vi "Initialization_HGB2.vi"(8 "error in":errorcluster, 11 "Sample Rate":dbl=10.0) -> (0 "error out":errorcluster, 3 "Task Array":refnum<k21>[](array[refnum]), 4 "output cluster":T1={"All Channels"=["cDAQ1Mod1/ai0", "cDAQ1Mod1/ai1", "cDAQ1Mod1/ai2", "cDAQ1Mod1/ai3", "cDAQ1Mod1/ai4", "cDAQ1Mod1/ai5", "cDAQ1Mod1/ai6", "cDAQ1Mod1/ai7", "cDAQ1Mod1/ai8", "cDAQ1Mod1/ai9", "cDAQ1Mod1/ai10", "cDAQ1Mod1/ai11", "cDAQ1Mod1/ai12", "cDAQ1Mod1/ai13", "cDAQ1Mod1/ai14", "cDAQ1Mod1/ai15", "cDAQ1Mod2/ai0", "cDAQ1Mod2/ai1", "cDAQ1Mod2/ai2", "cDAQ1Mod2/ai3", "cDAQ1Mod2/ai4", "cDAQ1Mod2/ai5", "cDAQ1Mod2/ai6", "cDAQ1Mod2/ai7", "cDAQ1Mod4/ai0", "cDAQ1Mod4/ai1", "cDAQ1Mod4/ai2", "Dev1/ai0", "Dev1/ai1", "Dev1/ao0", "Dev1/ao1"], "All Labels"=["T_dis", "T_liq_mix", "T_gas_mix", "T_wf_cond_out", "T_cf_in", "NC1", "NC2", "NC3", "NC4", "NC5", "NC6", "NC7", "NC8", "NC9", "NC10", "NC11", "P_comp_suc", "P_comp_dis", "P_comp_int", "m_dot_wf", "Voltage", "Frequency", "NC12", "NC13", "Accel_X", "Accel_Y", "Accel_Z", "Torque", "Tachometer", "Speed Setpoint", "ON-OFF"], "All Units"=["C", "C", "C", "C", "C", "C", "C", "C", "C", "C", "C", "C", "C", "C", "C", "C", "kPa", "kPa", "kPa", "kg/s", "V", "Hz", "A", "A", "g", "g", "g", "N-m", "RPM", "V", "V"], "Slope"=[1.0, 1.0, 1.0, 1.0, 1.0, 1.0, 1.0, 1.0, 1.0, 1.0, 1.0, 1.0, 1.0, 1.0, 1.0, 1.0, 129276.875, 129276.875, 129276.875, 4.6875, 18750.0, 6250.0, 5.0, 6250.0, 1.0, 1.0, 1.0, 4.0, 1600.0, 1.0, 1.0], "Y-Intercept"=[0.0, 0.0, 0.0, 0.0, 0.0, 0.0, 0.0, 0.0, 0.0, 0.0, 0.0, 0.0, 0.0, 0.0, 0.0, 0.0, -432.107, -435.107, -432.107, -0.01875, -75.0, -25.0, 0.0, 0.0, 0.0, 0.0, 0.0, 0.0, 0.0, 0.0, 0.0]})   [LabVIEW 2016]
uses:
  <vilib>/Utility/error.llb/DialogType.ctl
  <vilib>/DAQmx/create/channels.llb/DAQmx Create Channel (AI-Temperature-Thermocouple).vi
  <vilib>/DAQmx/create/scale.llb/DAQmx Create Scale (Linear).vi
  <vilib>/DAQmx/create/channels.llb/DAQmx Create Channel (AI-Voltage-Basic).vi
  <vilib>/DAQmx/create/channels.llb/DAQmx Create Channel (AO-Voltage-Basic).vi
  <vilib>/DAQmx/create/channels.llb/DAQmx Create Channel (AI-Current-Basic).vi
  <vilib>/DAQmx/create/channels.llb/DAQmx Create Channel (AO-Current-Basic).vi
  <vilib>/DAQmx/create/channels.llb/DAQmx Create Channel (AI-Acceleration-Accelerometer).vi
  <vilib>/DAQmx/configure/timing.llb/DAQmx Timing (Sample Clock).vi
panel:
  in  "Tab Control":enum32{"User Inputs", "Sub VI I/O"}(tab)
  in  "All Units":string[](array[string])=["C", "C", "C", "C", "C", "C", "C", "C", "C", "C", "C", "C", "C", "C", "C", "C", "Hz", "V", "kPa", "kPa", "kPa", "kg/s", "A", "A", "g", "g", "g", "N-m", "RPM", "V", "V"]
  in  "Number/Types of Channels per Task":string[][](table)=[["16", "0", "0", "0"], ["0", "0", "2", "0"], ["0", "0", "0", "2"], ["8", "0", "0", "0"], ["0", "0", "0", ""], ["0", "3", "0", ""], ["0", "0", "0", ""]]
  in  "All Channels":tag[](array[tag])=["cDAQ1Mod1/ai0", "cDAQ1Mod1/ai1", "cDAQ1Mod1/ai2", "cDAQ1Mod1/ai3", "cDAQ1Mod1/ai4", "cDAQ1Mod1/ai5", "cDAQ1Mod1/ai6", "cDAQ1Mod1/ai7", "cDAQ1Mod1/ai8", "cDAQ1Mod1/ai9", "cDAQ1Mod1/ai10", "cDAQ1Mod1/ai11", "cDAQ1Mod1/ai12", "cDAQ1Mod1/ai13", "cDAQ1Mod1/ai14", "cDAQ1Mod1/ai15", "cDAQ1Mod2/ai0", "cDAQ1Mod2/ai1", "cDAQ1Mod2/ai2", "cDAQ1Mod2/ai3", "cDAQ1Mod2/ai4", "cDAQ1Mod2/ai5", "cDAQ1Mod2/ai6", "cDAQ1Mod2/ai7", "cDAQ1Mod4/ai0", "cDAQ1Mod4/ai1", "cDAQ1Mod4/ai2", "Dev1/ai0", "Dev1/ai1", "Dev1/ao0", "Dev1/ao1"]
  in  "Task Count":i32=4
  in  "All Labels":string[](array[string])=["T_comp_suc", "T_comp_out", "NC1", "T_gas_mix", "T_wf_cd_out", "T_liq", "T_cf_in", "T_dis_dwnstrm", "NC2", "NC3", "NC4", "NC5", "NC6", "NC7", "NC8", "NC9", "Frequency", "Voltage", "P_comp_suc", "P_comp_dis", "P_comp_int", "m_dot_wf", "NC12", "NC13", "Accel_X", "Accel_Y", "Accel_Z", "Torque", "Tachometer", "Speed Setpoint", "ON-OFF"]
  in  "Y-Intercept":dbl[](array[numeric])=[0.0, 0.0, 0.0, 0.0, 0.0, 0.0, 0.0, 0.0, 0.0, 0.0, 0.0, 0.0, 0.0, 0.0, 0.0, 0.0, -25.0, -75.0, -432.107, -432.107, -432.107, -0.0225, 0.0, 0.0, 0.0, 0.0, 0.0, 0.0, 0.0, 0.0, 0.0]
  in  "Slope":dbl[](array[numeric])=[1.0, 1.0, 1.0, 1.0, 1.0, 1.0, 1.0, 1.0, 1.0, 1.0, 1.0, 1.0, 1.0, 1.0, 1.0, 1.0, 6250.0, 18750.0, 129276.875, 129277.0, 129277.0, 5.625, 5.0, 6250.0, 1.0, 1.0, 1.0, 4.0, 1600.0, 1.0, 1.0]
  # "*Make Current Values Default and Save Before Closing Sub VI*"
  # "*List the read and write channels of any hardware as separate devices*"
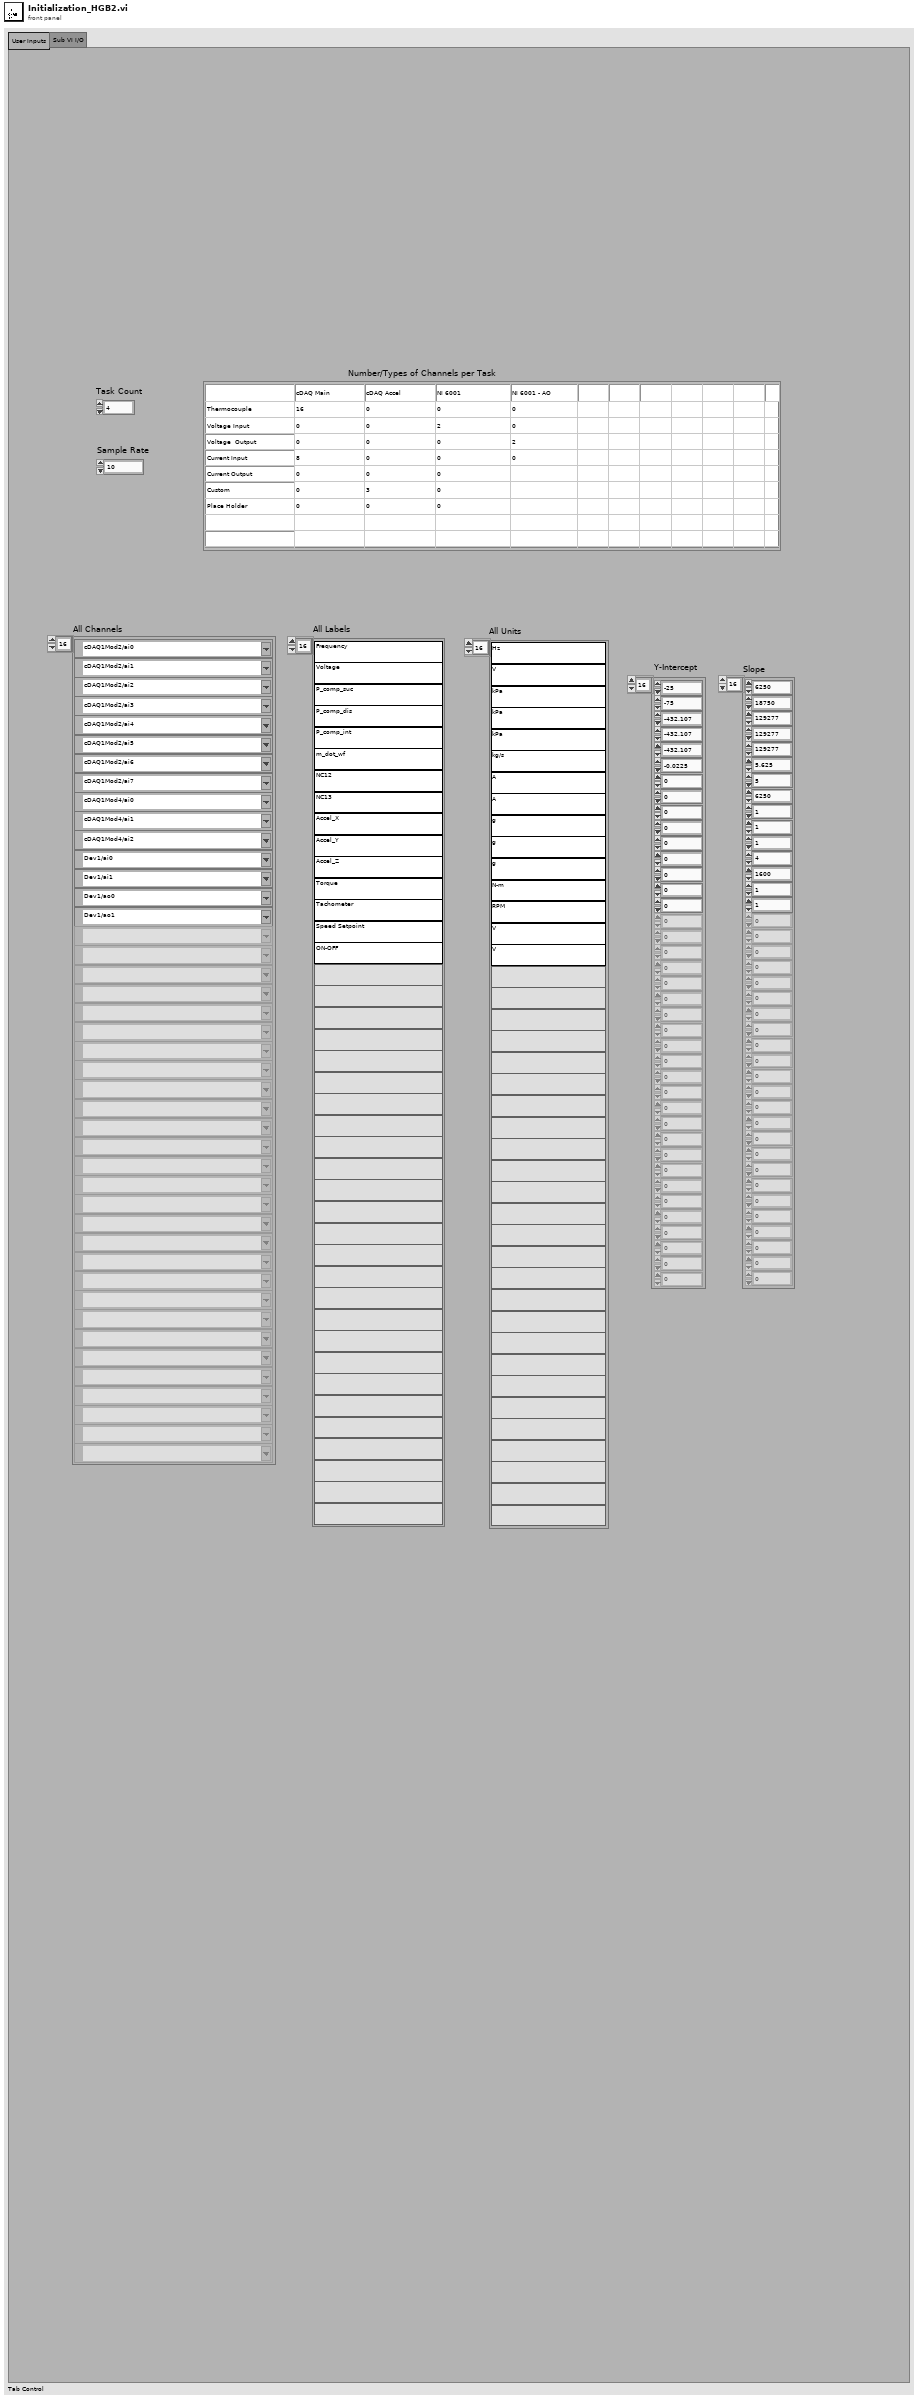
[diagram p1: front panel]
types:
  T1 = cluster{"All Channels":tag[], "All Labels":string[], "All Units":string[], "Slope":dbl[], "Y-Intercept":dbl[]}
  T2 = typedef "DialogType.ctl" = u16
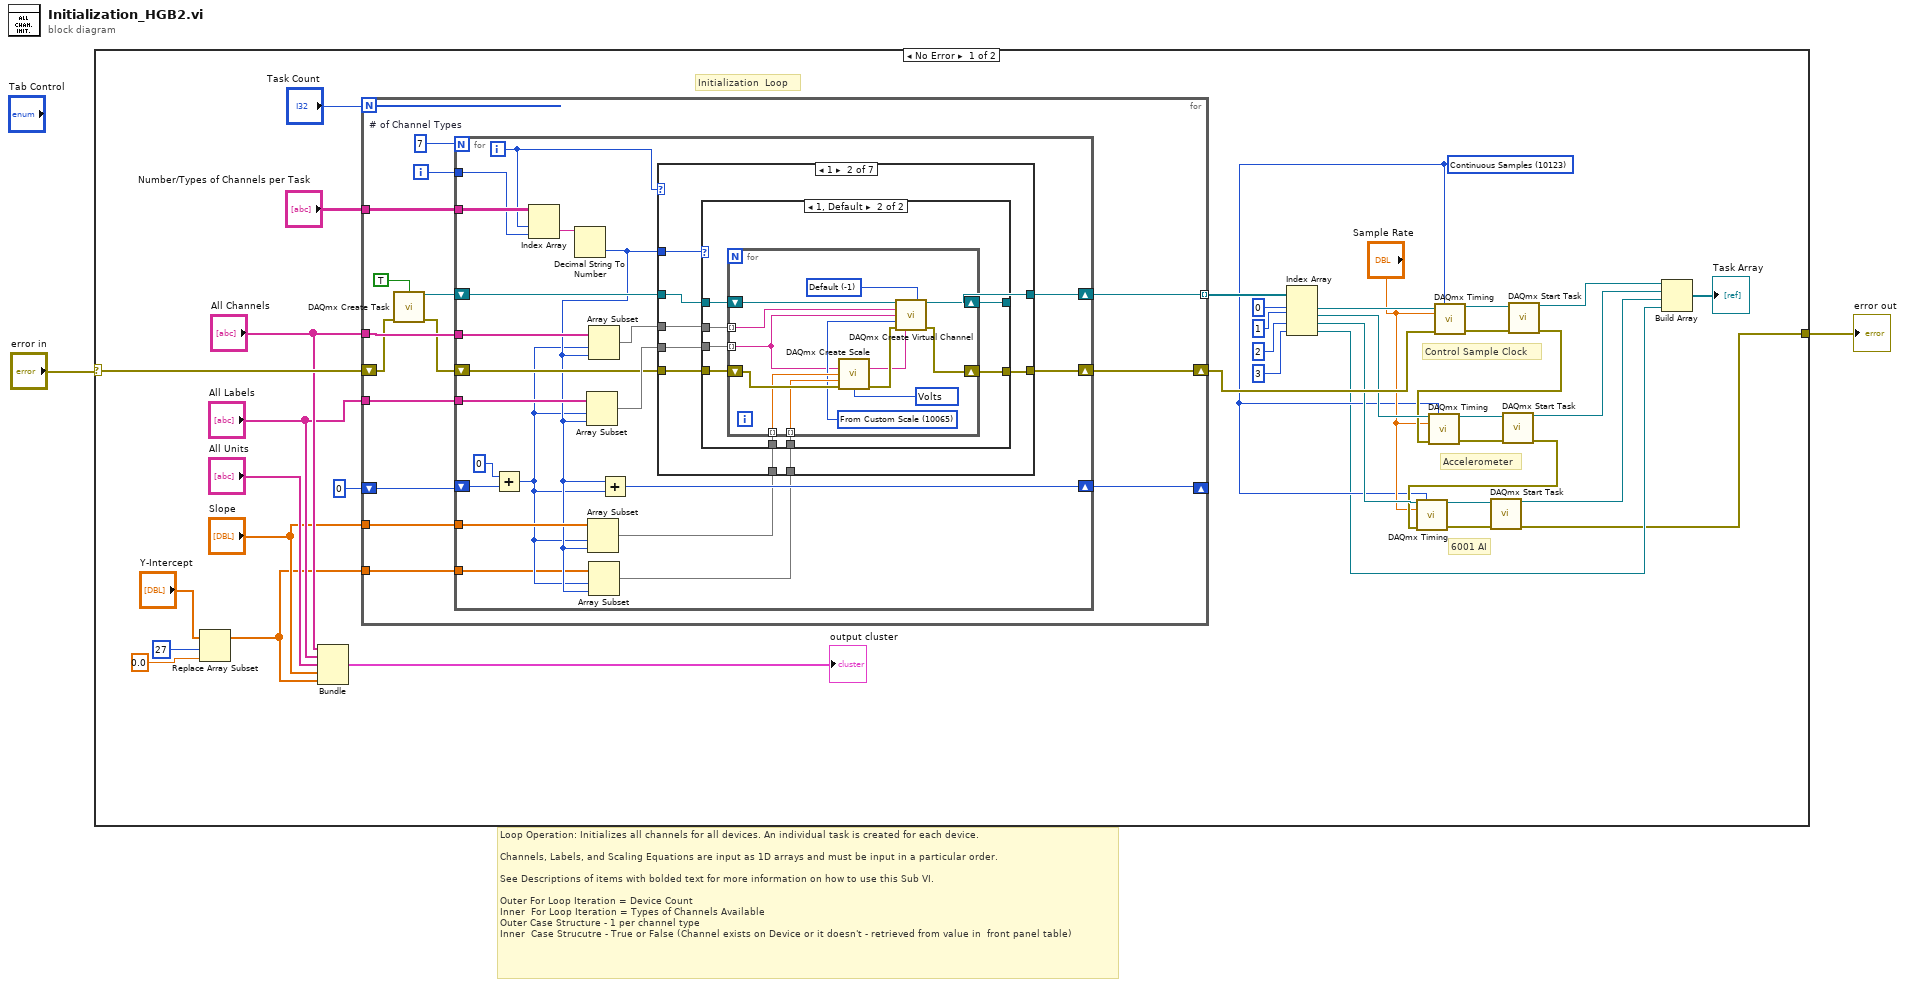
[diagram p0: block diagram]
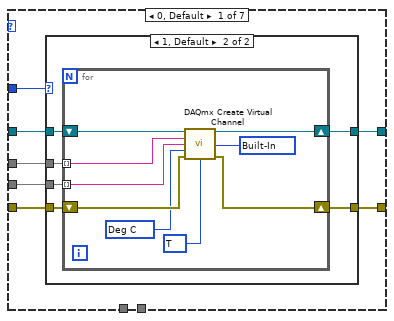
[diagram p2: hidden frame]
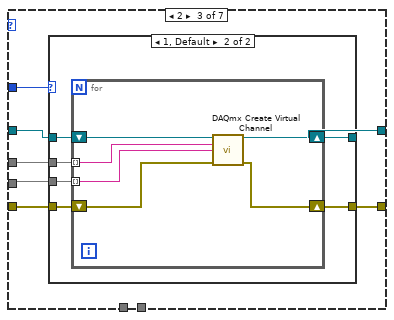
[diagram p5: hidden frame]
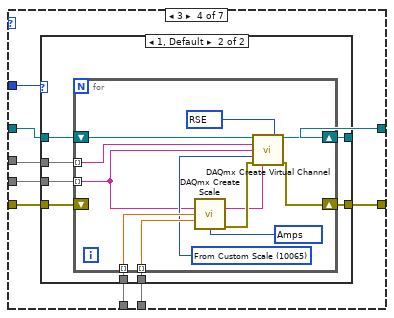
[diagram p7: hidden frame]
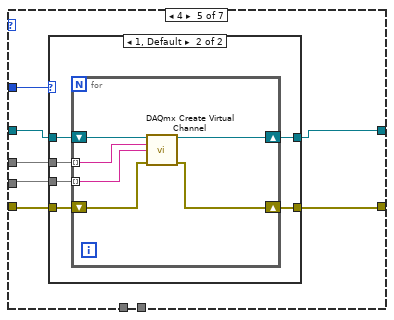
[diagram p9: hidden frame]
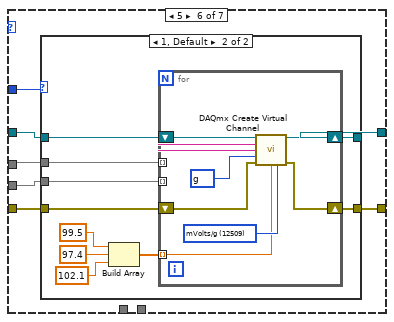
[diagram p11: hidden frame]
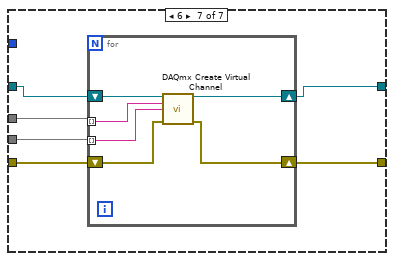
[diagram p13: hidden frame]
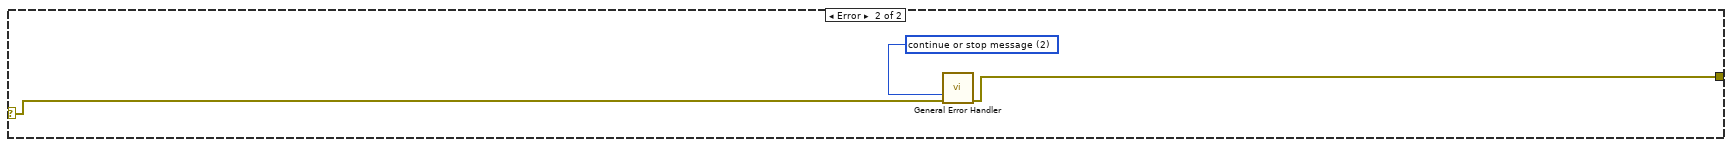
[diagram p14: hidden frame]
diagram:
  # "Loop Operation: Initializes all channels for all devices. An individual task is created for each device.\n\nChannels, Labels, and Scaling Equations are input as 1D arrays and must be input in a particular order.\n\nSee Descriptions of items with bolded text for more information on how to use this Sub VI.\n\nOuter For Loop Iteration = Device Count \nInner  For Loop Iteration = Types of Channels Available\nOuter Case Structure - 1 per channel type\nInner  Case Strucutre - True or False (Channel exists on Device or it doesn't - retrieved from value in  front panel table)"
  n1 = case shown="No Error" "error in" {
    selector: "error in" -> [w36 w247]
    tunnel: [w3 w246] -> w2
    frame No Error {
      w5 = 10123 items=["Finite Samples"=10178, "Continuous Samples"=10123, "Hardware Timed Single Point"=12522] ("sample mode")
      # "Accelerometer"
      # "6001 AI"
      # "Initialization  Loop"
      # "Control Sample Clock"
      n2 = Replace Array Subset(array="Y-Intercept", new element=0.0 ("new element/subarray"), index=27) -> (w20:dbl[])
      n3 = Bundle("All Channels"="All Channels", "All Labels"="All Labels", "All Units"="All Units", "Slope"="Slope", "Y-Intercept"=w20) -> (→"output cluster":T1)  [unwired: 1 in]
      n4 = for {
        N: "Task Count" -> [_]
        tunnel: "Number/Types of Channels per Task" -> [w55]
        tunnel: "All Channels" -> [w54]
        tunnel: "All Labels" -> [w53]
        shift-right: [w51] -> _
        shift-left: 0 -> [w50]
        tunnel: [w48] -> w32 mode=indexing
        shift-right: [w47] -> w37
        shift-left: w36 -> [w42]
        tunnel: "Slope" -> [w46]
        tunnel: w20 -> [w45]
        i -> [w52]
        w49 = 7  # # of Channel Types
        n5 = call <vilib>:"DAQmx Create Task.vi"("auto cleanup"=TRUE, "error in"=w42) -> ("task out"=w44:refnum<k21>, "error out"=w41:errorcluster)  [unwired: 12 in]
        n6 = for {
          N: w49 -> [_]
          tunnel: w55 -> [w75]
          tunnel: w54 -> [w74]
          tunnel: w53 -> [w73]
          tunnel: w52 -> [w56]
          shift-right: [w69] -> w51
          shift-left: w50 -> [w68]
          shift-right: [w66] -> w48
          shift-left: w44 -> [w65]
          shift-right: [w64] -> w47
          shift-left: w41 -> [w63]
          tunnel: w46 -> [w62]
          tunnel: w45 -> [w59]
          i -> [w67]
          n7 = Add(x=0 ("index"), y=w68) -> (x+y=w60:i32)
          n8 = Index Array(array=w75, index (row)=w67, index (col)=w56) -> (element=w76:string)
          n9 = Decimal String To Number(string=w76) -> (number=w61:i32)  [unwired: 2 in, 1 out]
          n10 = Array Subset(array=w73, index=w60, length=w61) -> (w71:string[])
          n11 = Array Subset(array=w62, index=w60, length=w61) -> (w58:dbl[])
          n12 = Array Subset(array=w74, index=w60, length=w61) -> (w72:tag[])
          n13 = Array Subset(array=w59, index=w60, length=w61) -> (w57:dbl[])
          n14 = Add(x=w61, y=w60) -> (x+y=w69:i32)
          n15 = case shown="1" w67 {
            tunnel: w72 -> [w83 w108 w138 w161 w190 w211 w239]
            tunnel: w71 -> [w82 w109 w139 w162 w191 w212 w238]
            tunnel: w61 -> [w81 w105 w135 w158 w187 w208 _]
            tunnel: [w80 w106 w136 w159 w188 w209 w235] -> w66
            tunnel: w65 -> [w79 w107 w137 w160 w189 w210 w234]
            tunnel: [w78 w104 w133 w156 w185 w206 w236] -> w64
            tunnel: w63 -> [w77 w103 w134 w157 w186 w207 w237]
            tunnel: w58 -> [_ w102 _ w155 _ _ _]
            tunnel: w57 -> [_ w101 _ w154 _ _ _]
            frame 0, Default {
              n16 = case shown="1, Default" w81 {
                tunnel: [w85 w91] -> w80
                tunnel: w83 -> [_ w90]
                tunnel: w82 -> [_ w89]
                tunnel: w79 -> [w85 w88]
                tunnel: [w84 w87] -> w78
                tunnel: w77 -> [w84 w86]
                frame 0 {
                }
                frame 1, Default {
                  n17 = for {
                    tunnel: w90 -> [w99] mode=indexing
                    tunnel: w89 -> [w98] mode=indexing
                    shift-right: [w100] -> w91
                    shift-left: w88 -> [w97]
                    shift-right: [w96] -> w87
                    shift-left: w86 -> [w95]
                    w92 = 10200 items=["Built-In"=10200, "Constant Value"=10116, "Channel"=10113] ("cjc source")
                    w93 = 10086 items=["J"=10072, "K"=10073, "N"=10077, "R"=10082, "S"=10085, "T"=10086, "B"=10047, "E"=10055] ("thermocouple type")
                    w94 = 10143 items=["Deg C"=10143, "Deg F"=10144, "Kelvins"=10325, "Deg R"=10145, "From Custom Scale"=10065] ("units")
                    n18 = call-poly <vilib>:"DAQmx Create Virtual Channel.vi"("task in"=w97, "physical channels"=w99, "cjc source"=w92, "name to assign"=w98, "units"=w94, "error in"=w95, "thermocouple type"=w93) -> ("task out"=w100:refnum<k21>, "error out"=w96:errorcluster)  [unwired: 7 in]
                  }
                }
              }
            }
            frame 1 {
              n19 = case shown="1, Default" w105 {
                tunnel: w107 -> [w111 w119]
                tunnel: [w111 w118] -> w106
                tunnel: w108 -> [_ w117]
                tunnel: w109 -> [_ w116]
                tunnel: [w110 w114] -> w104
                tunnel: w103 -> [w110 w115]
                tunnel: w102 -> [_ w113]
                tunnel: w101 -> [_ w112]
                frame 0 {
                }
                frame 1, Default {
                  n20 = for {
                    tunnel: w117 -> [w130] mode=indexing
                    tunnel: w116 -> [w120] mode=indexing
                    shift-right: [w131] -> w118
                    shift-left: w119 -> [w132]
                    shift-right: [w127] -> w114
                    shift-left: w115 -> [w129]
                    tunnel: w113 -> [w126] mode=indexing
                    tunnel: w112 -> [w125] mode=indexing
                    w122 = -1 items=["Default"=-1, "RSE"=10083, "NRSE"=10078, "Differential"=10106, "Pseudodifferential"=12529] ("input terminal configuration")
                    w123 = 10348 items=["Volts"=10348, "Amps"=10342, "Deg F"=10144, "Deg C"=10143, "Deg R"=10145, "Kelvins"=10325, "Strain"=10299, "Ohms"=10384, "Hz"=10373, "Seconds"=10364, "Meters"=10219, "Inches"=10379, "Degrees"=10146, "Radians"=10273, "Ticks"=10304, "g"=10186, "m/s^2"=12470, "m/s"=15959, "in/s"=15960, "Pascals"=10081, "Newtons"=15875, "Pounds"=15876, "kgf"=15877, "psi"=15879, "bar"=15880, "Nm"=15881, "oz-in"=15882, "lb-in"=15883, "lb-ft"=15884, "Volts/Volt"=15896, "mVolts/Volt"=15897, "From TEDS"=12516] ("pre-scaled units")
                    w124 = 10065 items=["Volts"=10348, "From Custom Scale"=10065] ("units")
                    n21 = call-poly <vilib>:"DAQmx Create Scale.vi"("name"=w120, "slope"=w126, "y-intercept"=w125, "error in"=w129, "pre-scaled units"=w123) -> ("scale out"=w121:tag, "error out"=w128:errorcluster)  [unwired: 9 in]
                    n22 = call-poly <vilib>:"DAQmx Create Virtual Channel.vi"("task in"=w132, "input terminal configuration"=w122, "physical channels"=w130, "name to assign"=w120, "units"=w124, "error in"=w128, "custom scale name"=w121) -> ("task out"=w131:refnum<k21>, "error out"=w127:errorcluster)  [unwired: 7 in]
                  }
                }
              }
            }
            frame 2 {
              n23 = case shown="1, Default" w135 {
                tunnel: w137 -> [w141 w147]
                tunnel: [w141 w146] -> w136
                tunnel: w138 -> [_ w145]
                tunnel: w139 -> [_ w144]
                tunnel: w134 -> [w140 w143]
                tunnel: [w140 w142] -> w133
                frame 0 {
                }
                frame 1, Default {
                  n24 = for {
                    tunnel: w145 -> [w151] mode=indexing
                    tunnel: w144 -> [w150] mode=indexing
                    shift-right: [w152] -> w146
                    shift-left: w147 -> [w153]
                    shift-right: [w148] -> w142
                    shift-left: w143 -> [w149]
                    n25 = call-poly <vilib>:"DAQmx Create Virtual Channel.vi"("task in"=w153, "physical channels"=w151, "name to assign"=w150, "error in"=w149) -> ("task out"=w152:refnum<k21>, "error out"=w148:errorcluster)  [unwired: 10 in]
                  }
                }
              }
            }
            frame 3 {
              n26 = case shown="1, Default" w158 {
                tunnel: w160 -> [w164 w172]
                tunnel: [w164 w171] -> w159
                tunnel: w161 -> [_ w170]
                tunnel: w162 -> [_ w169]
                tunnel: w157 -> [w163 w168]
                tunnel: [w163 w167] -> w156
                tunnel: w155 -> [_ w166]
                tunnel: w154 -> [_ w165]
                frame 0 {
                }
                frame 1, Default {
                  n27 = for {
                    tunnel: w170 -> [w182] mode=indexing
                    tunnel: w169 -> [w173] mode=indexing
                    shift-right: [w183] -> w171
                    shift-left: w172 -> [w184]
                    shift-right: [w181] -> w167
                    shift-left: w168 -> [_]
                    tunnel: w166 -> [w178] mode=indexing
                    tunnel: w165 -> [w177] mode=indexing
                    w174 = 10083 items=["default"=-1, "RSE"=10083, "NRSE"=10078, "Differential"=10106, "Pseudodifferential"=12529] ("input terminal configuration")
                    w176 = 10342 items=["Volts"=10348, "Amps"=10342, "Deg F"=10144, "Deg C"=10143, "Deg R"=10145, "Kelvins"=10325, "Strain"=10299, "Ohms"=10384, "Hz"=10373, "Seconds"=10364, "Meters"=10219, "Inches"=10379, "Degrees"=10146, "Radians"=10273, "Ticks"=10304, "g"=10186, "m/s^2"=12470, "m/s"=15959, "in/s"=15960, "Pascals"=10081, "Newtons"=15875, "Pounds"=15876, "kgf"=15877, "psi"=15879, "bar"=15880, "Nm"=15881, "oz-in"=15882, "lb-in"=15883, "lb-ft"=15884, "Volts/Volt"=15896, "mVolts/Volt"=15897, "From TEDS"=12516] ("pre-scaled units")
                    w175 = 10065 items=["Amps"=10342, "From Custom Scale"=10065] ("units")
                    n28 = call-poly <vilib>:"DAQmx Create Scale.vi"("name"=w173, "slope"=w178, "y-intercept"=w177, "pre-scaled units"=w176) -> ("scale out"=w179:tag, "error out"=w180:errorcluster)  [unwired: 10 in]
                    n29 = call-poly <vilib>:"DAQmx Create Virtual Channel.vi"("task in"=w184, "input terminal configuration"=w174, "physical channels"=w182, "name to assign"=w173, "units"=w175, "error in"=w180, "custom scale name"=w179) -> ("task out"=w183:refnum<k21>, "error out"=w181:errorcluster)  [unwired: 7 in]
                  }
                }
              }
            }
            frame 4 {
              n30 = case shown="1, Default" w187 {
                tunnel: w189 -> [w193 w199]
                tunnel: [w193 w198] -> w188
                tunnel: w190 -> [_ w197]
                tunnel: w191 -> [_ w196]
                tunnel: w186 -> [w192 w195]
                tunnel: [w192 w194] -> w185
                frame 0 {
                }
                frame 1, Default {
                  n31 = for {
                    tunnel: w197 -> [w203] mode=indexing
                    tunnel: w196 -> [w202] mode=indexing
                    shift-right: [w204] -> w198
                    shift-left: w199 -> [w205]
                    shift-right: [w201] -> w194
                    shift-left: w195 -> [w200]
                    n32 = call-poly <vilib>:"DAQmx Create Virtual Channel.vi"("task in"=w205, "physical channels"=w203, "name to assign"=w202, "error in"=w200) -> ("task out"=w204:refnum<k21>, "error out"=w201:errorcluster)  [unwired: 10 in]
                  }
                }
              }
            }
            frame 5 {
              n33 = case shown="1, Default" w208 {
                tunnel: w210 -> [w214 w223]
                tunnel: [w214 w224] -> w209
                tunnel: w211 -> [_ w220]
                tunnel: w212 -> [_ w219]
                tunnel: w207 -> [w213 w222]
                tunnel: [w213 w221] -> w206
                frame 0 {
                }
                frame 1, Default {
                  n34 = Build Array(99.5, 97.4, 102.1) -> (w215:dbl[])
                  n35 = for {
                    shift-right: [w233] -> w224
                    shift-left: w223 -> [w232]
                    shift-right: [w230] -> w221
                    shift-left: w222 -> [w231]
                    tunnel: w220 -> [w229] mode=indexing
                    tunnel: w219 -> [w228] mode=indexing
                    tunnel: w215 -> [w225] mode=indexing
                    w226 = 12509 items=["mVolts/g"=12509, "Volts/g"=12510] ("sensitivity units")
                    w227 = 10186 items=["g"=10186, "m/s^2"=12470, "in/s^2"=12471, "From Custom Scale"=10065] ("units")
                    n36 = call-poly <vilib>:"DAQmx Create Virtual Channel.vi"("task in"=w232, "physical channels"=w229, "name to assign"=w228, "units"=w227, "error in"=w231, "sensitivity"=w225, "sensitivity units"=w226) -> ("task out"=w233:refnum<k21>, "error out"=w230:errorcluster)  [unwired: 7 in]
                  }
                }
              }
            }
            frame 6 {
              n37 = for {
                tunnel: w239 -> [w243] mode=indexing
                tunnel: w238 -> [w242] mode=indexing
                shift-right: [w244] -> w235
                shift-left: w234 -> [w245]
                shift-right: [w241] -> w236
                shift-left: w237 -> [w240]
                n38 = call-poly <vilib>:"DAQmx Create Virtual Channel.vi"("task in"=w245, "physical channels"=w243, "name to assign"=w242, "error in"=w240) -> ("task out"=w244:refnum<k21>, "error out"=w241:errorcluster)  [unwired: 10 in]
              }
            }
          }
        }
      }
      n39 = Index Array(array=w32, index #1=0 ("index"), index #2=1 ("index"), index #3=2 ("index"), index #4=3 ("index")) -> (element #1=w38:refnum<k21>, element #2=w12:refnum<k21>, element #3=w13:refnum<k21>, element #4=w4:refnum<k21>)
      n40 = call-poly <vilib>:"DAQmx Timing.vi"("task/channels in"=w38, "sample mode"=w5, "rate"="Sample Rate", "error in"=w37) -> ("task out"=w35:refnum<k21>, "error out"=w34:errorcluster)  [unwired: 10 in]
      n41 = call <vilib>:"DAQmx Start Task.vi"("task/channels in"=w35, "error in"=w34) -> ("task out"=w31:refnum<k21>, "error out"=w11:errorcluster)  [unwired: 12 in]
      n42 = call-poly <vilib>:"DAQmx Timing.vi"("task/channels in"=w12, "sample mode"=w5, "rate"="Sample Rate", "error in"=w11) -> ("task out"=w16:refnum<k21>, "error out"=w15:errorcluster)  [unwired: 10 in]
      n43 = call <vilib>:"DAQmx Start Task.vi"("task/channels in"=w16, "error in"=w15) -> ("task out"=w8:refnum<k21>, "error out"=w10:errorcluster)  [unwired: 12 in]
      n44 = call-poly <vilib>:"DAQmx Timing.vi"("task/channels in"=w13, "sample mode"=w5, "rate"="Sample Rate", "error in"=w10) -> ("task out"=w19:refnum<k21>, "error out"=w18:errorcluster)  [unwired: 10 in]
      n45 = call <vilib>:"DAQmx Start Task.vi"("task/channels in"=w19, "error in"=w18) -> ("task out"=w9:refnum<k21>, "error out"=w3:errorcluster)  [unwired: 12 in]
      n46 = Build Array(w31, w8, w9, w4) -> (→"Task Array":refnum<k21>[])
    }
    frame Error {
      w248 = T2 2 items=["no dialog", "OK message", "continue or stop message", "OK message + warnings", "continue/stop + warnings"] ("type of dialog (OK msg:1)")
      n47 = call <vilib>:"General Error Handler.vi"("type of dialog (OK msg:1)"=w248, "error in (no error)"=w247) -> ("error out"=w246:errorcluster)  [unwired: 9 in, 4 out]
    }
  }
  "error out" <- w2
